vi "ParseSensors.vi"(0 "data out":string) -> (4 "x1":sgl, 6 "x2":sgl, 8 "x3":sgl, 9 "xa2":sgl, 10 "x4":sgl, 11 "x8":sgl, 12 "x7":sgl, 13 "x6":sgl, 14 "x5":sgl, 15 "xa1":sgl)   [LabVIEW 2009]
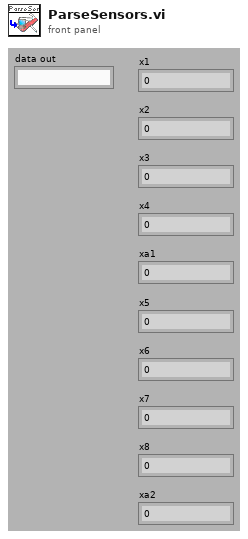
[diagram p1: front panel]
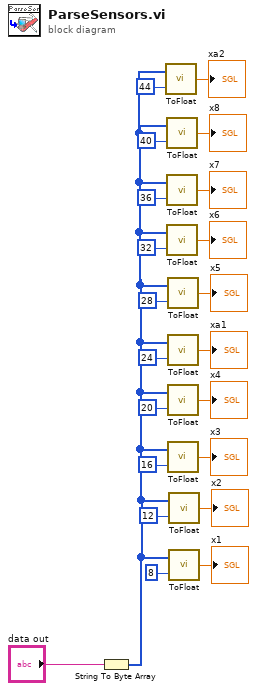
[diagram p0: block diagram]
diagram:
  n1 = String To Byte Array(string="data out") -> (unsigned byte array=w1:u8[])
  n2 = call "ToFloat.vi"("index"=44, "array"=w1) -> ("sp float"=→"xa2":sgl)
  n3 = call "ToFloat.vi"("index"=40, "array"=w1) -> ("sp float"=→"x8":sgl)
  n4 = call "ToFloat.vi"("index"=36, "array"=w1) -> ("sp float"=→"x7":sgl)
  n5 = call "ToFloat.vi"("index"=32, "array"=w1) -> ("sp float"=→"x6":sgl)
  n6 = call "ToFloat.vi"("index"=28, "array"=w1) -> ("sp float"=→"x5":sgl)
  n7 = call "ToFloat.vi"("index"=24, "array"=w1) -> ("sp float"=→"xa1":sgl)
  n8 = call "ToFloat.vi"("index"=20, "array"=w1) -> ("sp float"=→"x4":sgl)
  n9 = call "ToFloat.vi"("index"=16, "array"=w1) -> ("sp float"=→"x3":sgl)
  n10 = call "ToFloat.vi"("index"=12, "array"=w1) -> ("sp float"=→"x2":sgl)
  n11 = call "ToFloat.vi"("index"=8, "array"=w1) -> ("sp float"=→"x1":sgl)
